vi "Enable Authorized Controls.vi"(8 "error in (no error)":errorcluster, 11 "Authorized":T1) -> (0 "error out":errorcluster)   [LabVIEW 2020]
doc: "Author: Scott Hannahs <sth@magnet.fsu.edu>\nCopyright 2018 Florida State University, All rights reserved."
uses:
  SCM4 Interlock LV20/RT SubVIs/RT System Auth Level.ctl
  Interlock 32T Net Client Globals.vi
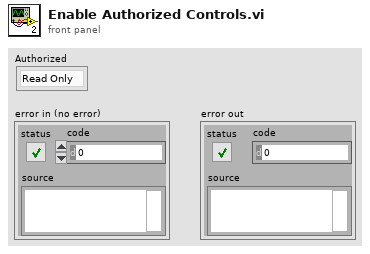
[diagram p1: front panel]
types:
  T1 = typedef "RT System Auth Level.ctl" = enum16{"Read Only", "User", "Operator", "Admin"}
  T2 = enum8{"Enabled", "Disabled", "Disabled and Grayed Out"}
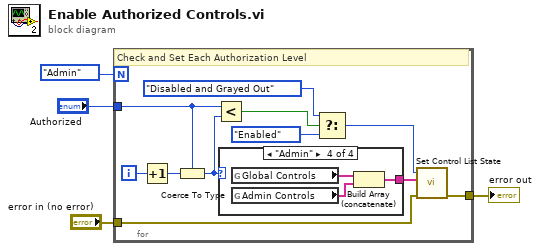
[diagram p0: block diagram]
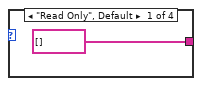
[diagram p2: hidden frame]
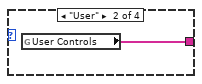
[diagram p3: hidden frame]
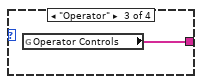
[diagram p4: hidden frame]
diagram:
  n1 = for {
    N: RT_System_Auth_Level."Admin" ("y") -> [_]
    tunnel: "Authorized" -> [w13]
    tunnel: [w7] -> w2
    tunnel: "error in (no error)" -> [w6]
    i -> [w15]
    # "Check and Set Each Authorization Level"
    n2 = Increment(x=w15) -> (x+1=w14:i32)
    n3 = Coerce To Type(0:w14, 1:w13) -> (2:w11:T1)
    n4 = Less?(x=w13, y=w11) -> (x < y?=w12:bool)
    n5 = case shown="\"Admin\"" w11 {
      tunnel: [string[] [] ("Operator Controls") w17 w18 w19] -> w8
      frame "Read Only", Default {
      }
      frame "User" {
        n6 = global read "Interlock 32T Net Client Globals.vi" "User Controls"() -> (w17:string[])
      }
      frame "Operator" {
        n7 = global read "Interlock 32T Net Client Globals.vi" "Operator Controls"() -> (w18:string[])
      }
      frame "Admin" {
        n8 = global read "Interlock 32T Net Client Globals.vi" "Global Controls"() -> (w21:string[])
        n9 = global read "Interlock 32T Net Client Globals.vi" "Admin Controls"() -> (w20:string[])
        n10 = Build Array (concatenate)(w21, w20) -> (w19:string[])
      }
    }
    n11 = Select(t=T2."Disabled and Grayed Out" ("Disabled"), s=w12, f=T2."Enabled" ("Disabled")) -> (s? t:f=w5:T2)
    n12 = call "Set Control List State.vi"("error in (no error)"=w6, "Control List"=w8, "Enable Disable"=w5) -> ("error out"=w7:errorcluster)  [unwired: 8 in]
  }
  "error out" <- w2
